vi "LuaVIEW Run or Swap Task_srv.vi"(0 "script file or name (no name)":path, 5 "action":enum16{"run", "swap"}(ring), 7 "certificate":string, 9 "identifier (use keyword)":string, 11 "script string (\"\" == load from file)":string) -> (4 "manual error":bool, 8 "identifier":string, 15 "error out":errorcluster)   [LabVIEW 2012]
doc: "Runs a new LuaVIEW task. This launches a task and waits until the task has progressed beyond its initialization. When the task fails while initializing, an error is returned."
uses:
  clientsrv/typedefs/t_ClientSrv Access Levels.ctl
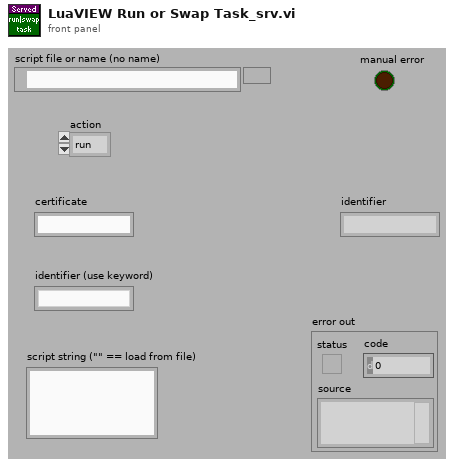
[diagram p1: front panel]
types:
  T1 = typedef "t_ClientSrv Access Levels.ctl" = enum16{"observer", "operator", "local"}
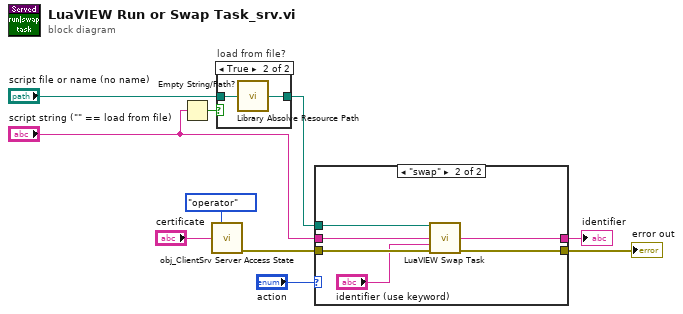
[diagram p0: block diagram]
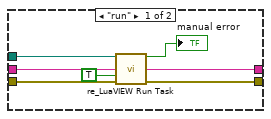
[diagram p3: hidden frame]
diagram:
  n1 = Empty String/Path?(string/path="script string (\"\" == load from file)") -> (empty?=w1:bool)
  n2 = call "obj_ClientSrv Server Access State.vi"("access level"=t_ClientSrv_Access_Levels."operator", "certificate in"="certificate") -> ("error out"=w8:errorcluster)  [unwired: 11 in, 2 out]
  n3 = case "load from file?" shown="True" w1 {
    tunnel: "script file or name (no name)" -> [w11 w13]
    tunnel: [w11 w12] -> w2
    frame False {
    }
    frame True {
      n4 = call "Library Absolve Resource Path.vi"("path in"=w13) -> ("absolved path"=w12:path)  [unwired: 14 in]
    }
  }
  n5 = case shown="\"swap\"" "action" {
    tunnel: [w20 w26] -> w10
    tunnel: w8 -> [w19 w25]
    tunnel: "script string (\"\" == load from file)" -> [w18 w24]
    tunnel: w2 -> [w17 w23]
    tunnel: [w16 w22] -> w6
    frame "run" {
      n6 = call "re_LuaVIEW Run Task.vi"("script file or name (no name)"=w17, "script string (\"\" == load from file)"=w18, "manual? (false)"=TRUE, "error in (no error)"=w19) -> ("manual error"=→"manual error":bool, "identifier"=w16:string, "error out"=w20:errorcluster)  [unwired: 9 in]
    }
    frame "swap" {
      n7 = call "LuaVIEW Swap Task.vi"("script file or name (no name)"=w23, "script string (\"\" == load from file)"=w24, "identifier (use keyword)"="identifier (use keyword)", "error in (no error)"=w25) -> ("identifier"=w22:string, "error out"=w26:errorcluster)  [unwired: 10 in]
    }
  }
  "error out" <- w10
  "identifier" <- w6
